vi "Apply min Threshold.vi"(8 "error in":errorcluster, 10 "Min. Thresh.":sgl, 11 "Image In":T1) -> (0 "error out":errorcluster, 3 "Image Out":T1)   [LabVIEW 2020, in "POLARIS Vision utility.lvlib"]
uses:
  POLARIS Vision utility.lvlib
  <vilib>/vision/Image Controls.llb/IMAQ Image.ctl
  <vilib>/vision/NI_Vision_Development_Module.lvlib
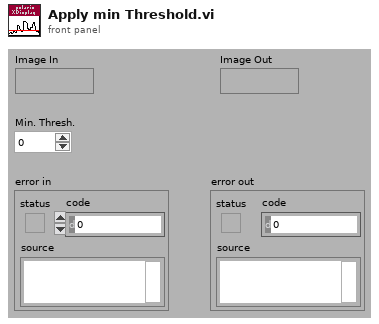
[diagram p1: front panel]
types:
  T1 = typedef "IMAQ Image.ctl" = refnum<image>
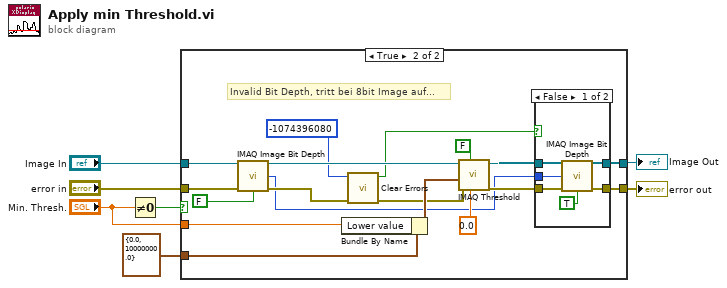
[diagram p0: block diagram]
diagram:
  n1 = Not Equal To 0?(x="Min. Thresh.") -> (x != 0?=w5:bool)
  n2 = case shown="True" w5 {
    tunnel: [w8 w27] -> w1
    tunnel: "Min. Thresh." -> [_ w26]
    tunnel: "Image In" -> [w9 w19]
    tunnel: "error in" -> [w8 w18]
    tunnel: [w9 w25] -> w3
    tunnel: cluster{"Lower value":sgl, "Upper value":sgl} {"Lower value"=0.0, "Upper value"=10000000.0} ("Tresh") -> [_ w14]
    frame False {
    }
    frame True {
      # "Invalid Bit Depth, tritt bei 8bit Image auf..."
      n3 = call "IMAQ Image Bit Depth"("Image"=w19, "error in (no error)"=w18, "Get/Set Bit Depth? (Set)"=FALSE) -> ("Image Out"=w15:T1, "Bit Depth"=w16:u32, "error out"=w17:errorcluster)  [unwired: 10 in]
      n4 = Bundle By Name(cluster=w14, "Lower value"=w26) -> (w22:cluster{"Lower value":sgl, "Upper value":sgl})
      n5 = call <vilib>:"Clear Errors.vi"("error in (no error)"=w17, "specific error code to clear (0: all)"=-1074396080) -> ("error out"=w12:errorcluster, "specific error cleared?"=w10:bool)  [unwired: 4 in]
      n6 = call "IMAQ Threshold"("Replace Value"=sgl 0.0, "Keep/Replace Value (Replace)"=FALSE, "error in (no error)"=w12, "Range"=w22, "Image Src"=w15) -> ("error out"=w20:errorcluster, "Image Dst Out"=w21:T1)  [unwired: 5 in]
      n7 = case shown="False" w10 {
        tunnel: [w33 w34] -> w27
        tunnel: [w32 w35] -> w25
        tunnel: w21 -> [w31 w35]
        tunnel: w20 -> [w30 w34]
        tunnel: w16 -> [w29 _]
        frame False {
          n8 = call "IMAQ Image Bit Depth"("Image"=w31, "Bit Depth (0)"=w29, "error in (no error)"=w30, "Get/Set Bit Depth? (Set)"=TRUE) -> ("Image Out"=w32:T1, "error out"=w33:errorcluster)  [unwired: 9 in, 1 out]
        }
        frame True {
        }
      }
    }
  }
  "Image Out" <- w3
  "error out" <- w1
